vi "PressureControl - 4He.vi"(8 "error in (no error)":errorcluster, 11 "VISA resource name":refnum<visa-resource-name>) -> (0 "error out":errorcluster, 1 "Pressure":dbl, 2 "Pressure (Torr)":string, 3 "VISA resource name out":refnum<visa-resource-name>)   [LabVIEW 2018]
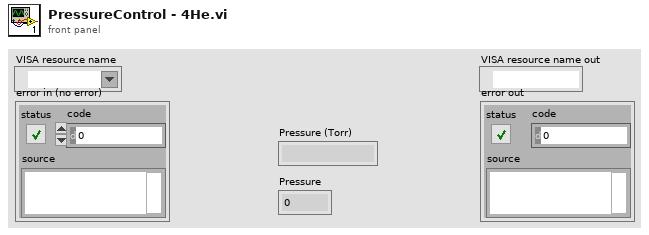
[diagram p1: front panel]
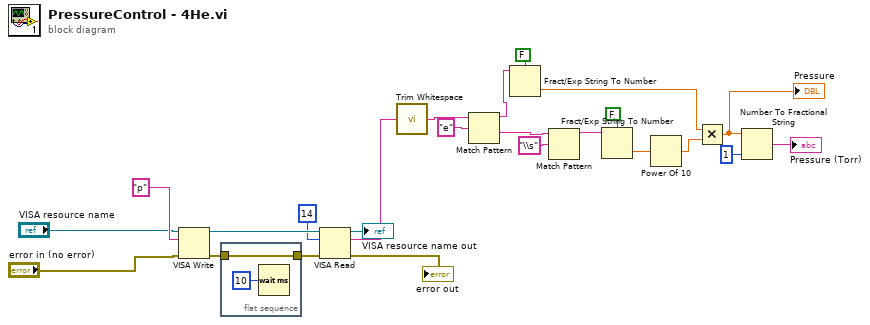
[diagram p0: block diagram]
diagram:
  n1 = VISA Write(VISA resource name="VISA resource name", write buffer="p", error in (no error)="error in (no error)") -> (VISA resource name out=w23:refnum<visa-resource-name>, error out=w24:errorcluster)  [unwired: 1 out]
  n2 = flat-sequence {
    tunnel: w24 -> [w25]
    tunnel: [w25] -> w22
    frame #0 {
      n3 = Wait (ms)(milliseconds to wait=u32 10) -> ()  [unwired: 1 out]
    }
  }
  n4 = VISA Read(VISA resource name=w23, byte count=u32 14, error in (no error)=w22) -> (VISA resource name out=→"VISA resource name out":refnum<visa-resource-name>, read buffer=w20:string, error out=→"error out":errorcluster)  [unwired: 1 out]
  n5 = call <vilib>:"Trim Whitespace.vi"("string"=w20) -> ("trimmed string"=w19:string)  [unwired: 1 in]
  n6 = Match Pattern(string=w19, regular expression="e") -> (before substring=w15:string, after substring=w14:string)  [unwired: 1 in, 2 out]
  n7 = Fract/Exp String To Number(use system decimal point (T)=FALSE, string=w15) -> (number=w10:dbl)  [unwired: 2 in, 1 out]
  n8 = Match Pattern(string=w14, regular expression="\\s") -> (before substring=w12:string)  [unwired: 1 in, 3 out]
  n9 = Fract/Exp String To Number(use system decimal point (T)=FALSE, string=w12) -> (number=w11:dbl)  [unwired: 2 in, 1 out]
  n10 = Power Of 10(x=w11) -> (10^x=w9:dbl)
  n11 = Multiply(x=w10, y=w9) -> (x*y=w8:dbl)
  "Pressure" <- w8
  n12 = Number To Fractional String(number=w8, precision (6)=i16 1) -> (F-format string=→"Pressure (Torr)":string)  [unwired: 2 in]
